vi "Untitled [Tset].vi"() -> ()   [LabVIEW 2012]
uses:
  <vilib>/Analysis/baseanly.llb/Real Dot Product.vi
  <vilib>/Analysis/NI_AALBase.lvlib
panel:
  out "XY Graph":cluster{"Y":dbl[], "Y":dbl[]}[](graph)
  out "Waveform Chart 5":dynamicdata(graph)
  out "Waveform Chart 4":dbl[](graph)
  out "output array":dbl[](array[numeric])
  out "Waveform Chart 3":dbl(graph)
  out "Waveform Chart 2":dynamicdata(graph)
  out "X速率(cm/s)":dbl
  out "Waveform Chart":dbl(graph)
  in  "退出程序":bool caption="停止电机 2"
  out "x/y":dbl
  out "Y偏移量 (cm)":dbl
  out "X偏移量 (cm)":dbl
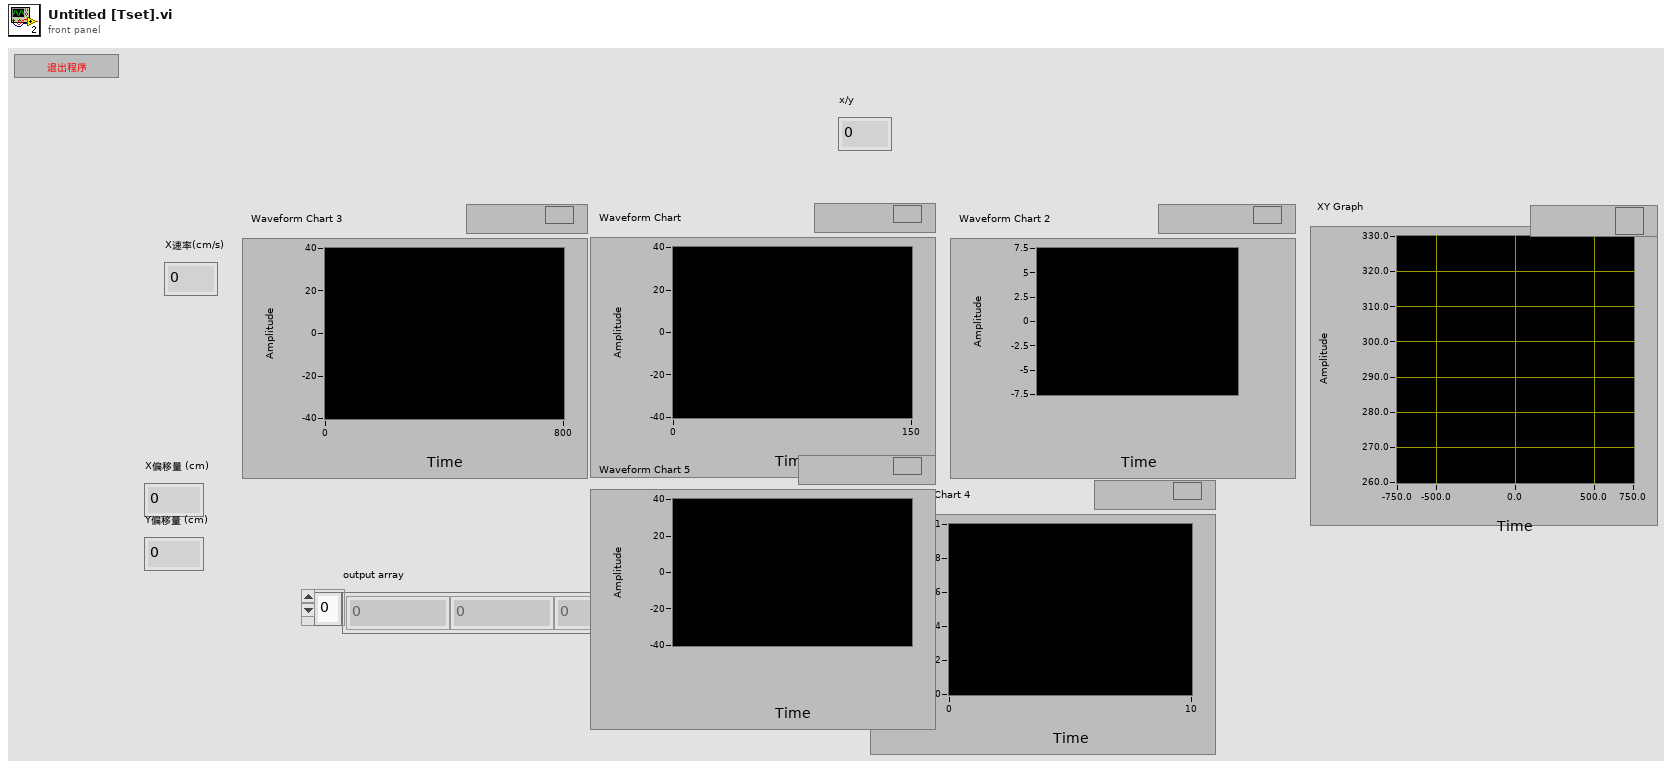
[diagram p1: front panel]
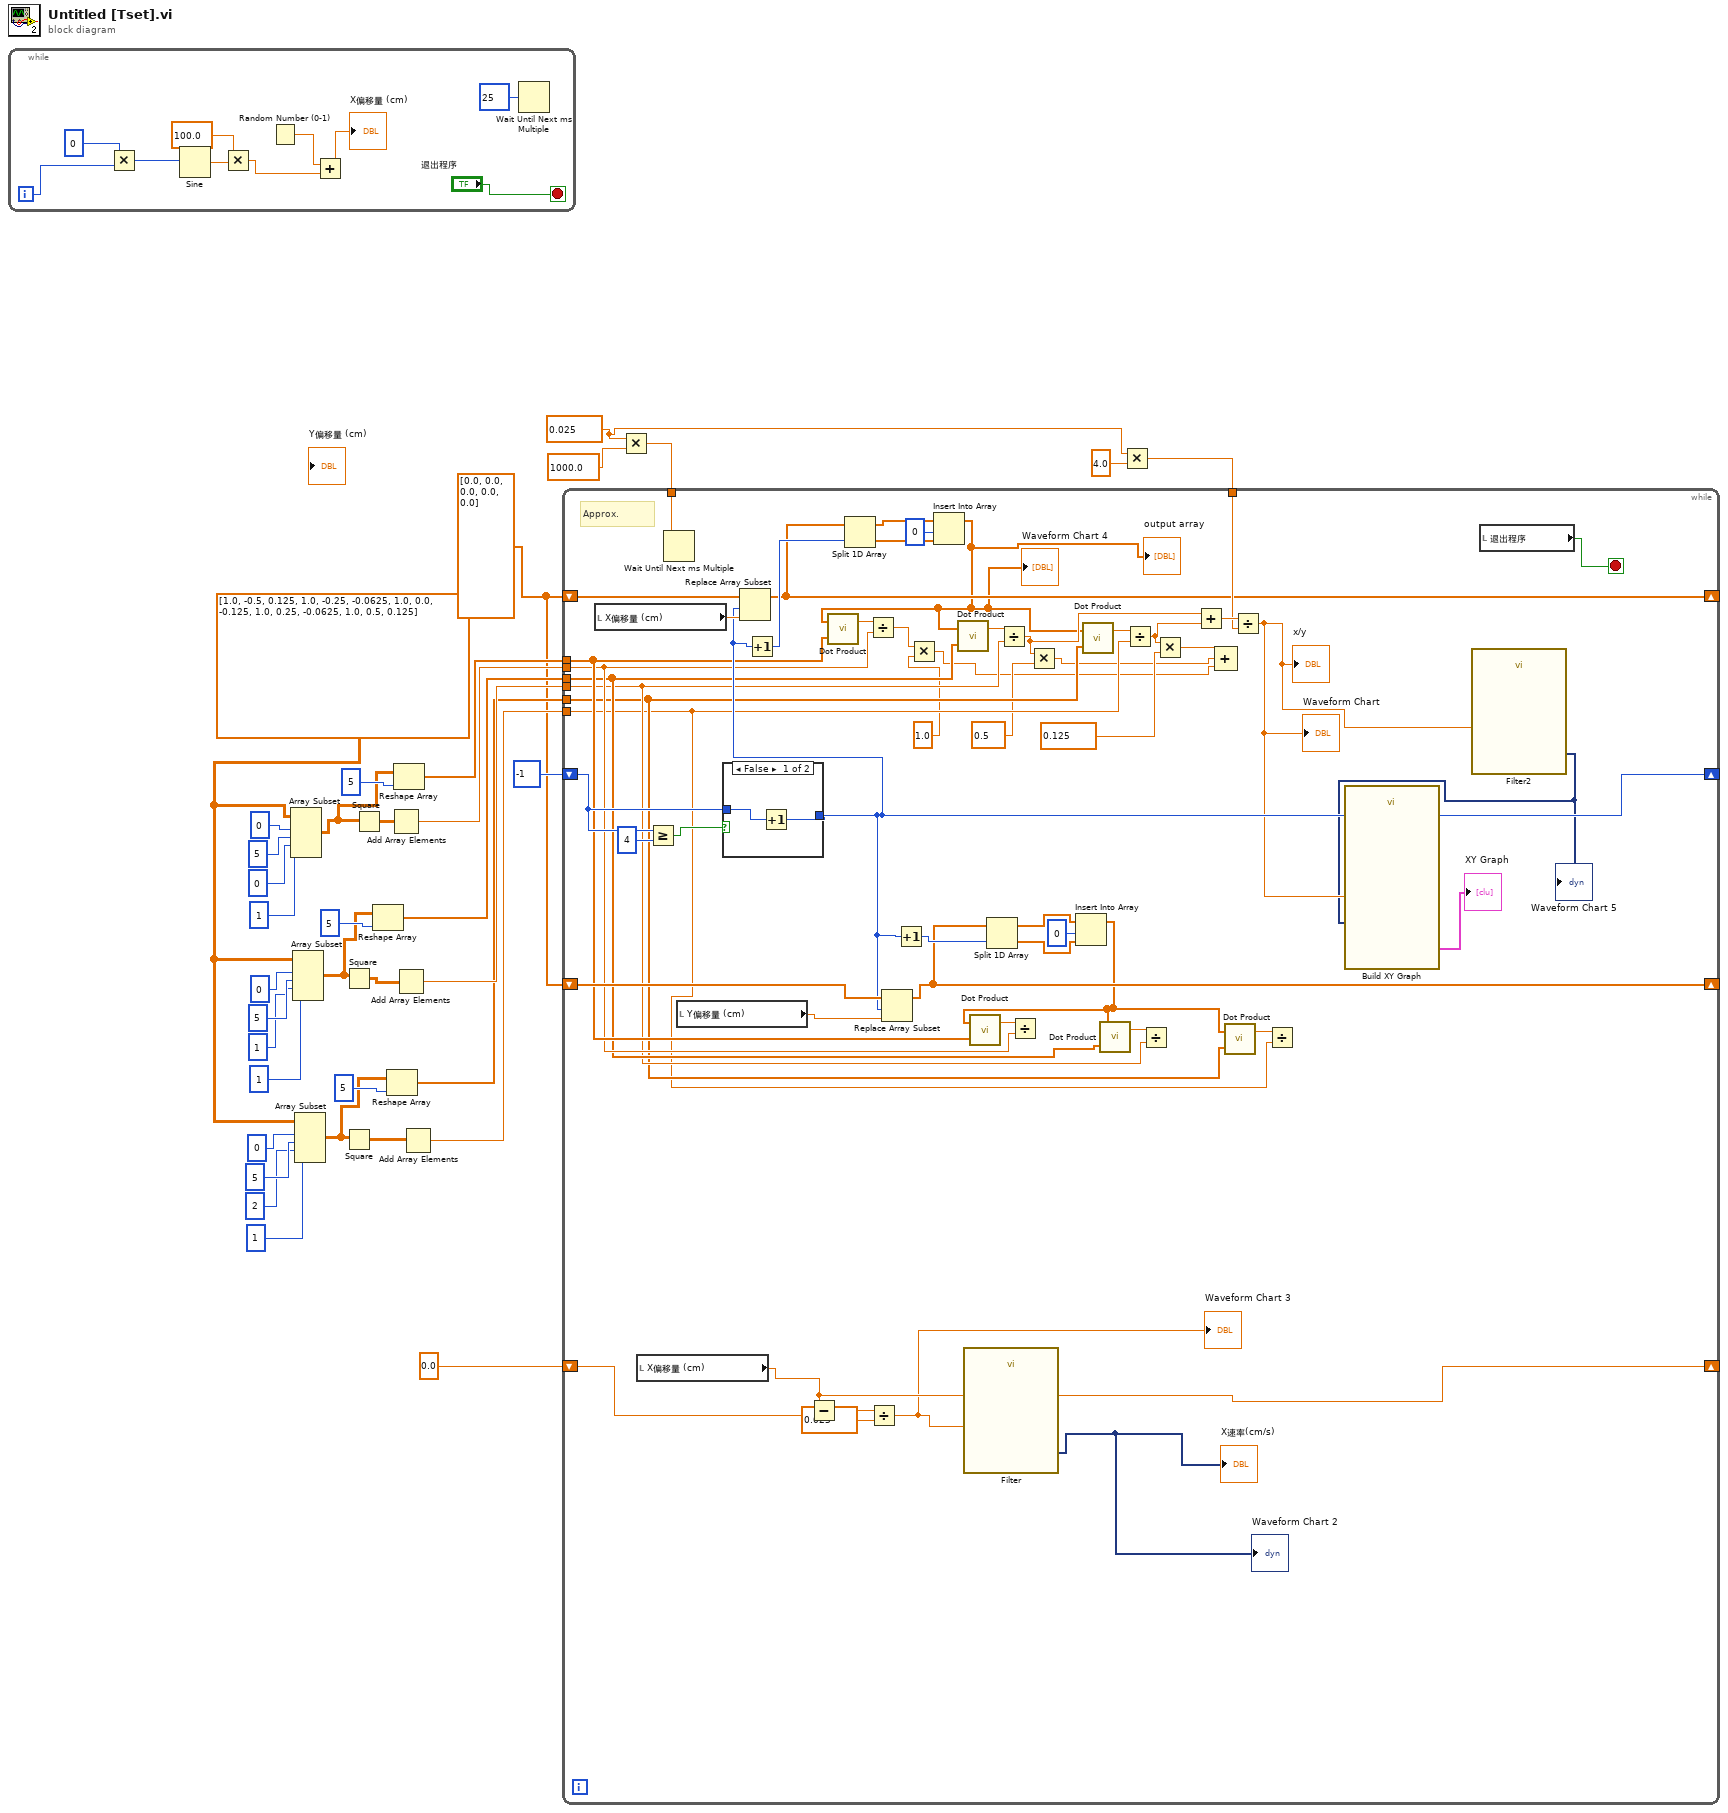
[diagram p0: block diagram]
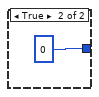
[diagram p2: hidden frame]
diagram:
  w3 = 0.025
  w20 = dbl[][] [[1.0, -0.5, 0.125], [1.0, -0.25, -0.0625], [1.0, 0.0, -0.125], [1.0, 0.25, -0.0625], [1.0, 0.5, 0.125]]
  w7 = dbl[] [0.0, 0.0, 0.0, 0.0, 0.0]
  n1 = while {
    i -> [w43]
    stop <- "退出程序" stop-if-true
    n2 = Multiply(x=0, y=w43) -> (x*y=w40:i32)
    n3 = Sine(x=w40) -> (sin(x)=w39:dbl)
    n4 = Multiply(x=100.0, y=w39) -> (x*y=w37:dbl)
    n5 = Random Number (0-1)() -> (number: 0 to 1=w44:dbl)
    n6 = Add(x=w44, y=w37) -> (x+y=→"X偏移量 (cm)":dbl)
    n7 = Wait Until Next ms Multiple(millisecond multiple=u32 25) -> ()  [unwired: 1 out]
  }
  n8 = Array Subset(array=w20, index (row)=0 ("index"), length (row)=5 ("length"), index (col)=0 ("index"), length (col)=1 ("length")) -> (w18:dbl[][])
  n9 = Array Subset(array=w20, index (row)=0 ("index"), length (row)=5 ("length"), index (col)=1 ("index"), length (col)=1 ("length")) -> (w14:dbl[][])
  n10 = Array Subset(array=w20, index (row)=0 ("index"), length (row)=5 ("length"), index (col)=2 ("index"), length (col)=1 ("length")) -> (w10:dbl[][])
  n11 = Square(x=w14) -> (x^2=w22:dbl[][])
  n12 = Square(x=w10) -> (x^2=w21:dbl[][])
  n13 = Square(x=w18) -> (x^2=w23:dbl[][])
  n14 = Reshape Array(w14, 5 ("dimension size")) -> (w13:dbl[])
  n15 = Reshape Array(w10, 5 ("dimension size")) -> (w9:dbl[])
  n16 = Add Array Elements(numeric array=w23) -> (sum=w16:dbl)
  n17 = Reshape Array(w18, 5 ("dimension size")) -> (w17:dbl[])
  n18 = Add Array Elements(numeric array=w22) -> (sum=w12:dbl)
  n19 = Add Array Elements(numeric array=w21) -> (sum=w8:dbl)
  n20 = Multiply(x=w3, y=1000.0) -> (x*y=w5:dbl)
  n21 = Multiply(x=w3, y=4.0) -> (x*y=w1:dbl)
  n22 = while {
    shift-right: [w51] -> _
    shift-left: w7 -> [w99]
    shift-right: [w85] -> _
    shift-left: -1 -> [w95]
    tunnel: w17 -> [w78]
    tunnel: w16 -> [w77]
    tunnel: w13 -> [w76]
    tunnel: w12 -> [w74]
    tunnel: w9 -> [w72]
    tunnel: w8 -> [w71]
    shift-right: [w83] -> _
    shift-left: w7 -> [w86]
    tunnel: w5 -> [w59]
    tunnel: w1 -> [w58]
    shift-right: [w55] -> _
    shift-left: 0.0 -> [w56]
    stop <- w100 stop-if-true
    # "Approx."
    n23 = local read "X偏移量 (cm)"() -> (w98:dbl)
    n24 = local read "X偏移量 (cm)"() -> (w55:dbl)
    n25 = Greater Or Equal?(x=w95, y=4) -> (x >= y?=w96:bool)
    n26 = Wait Until Next ms Multiple(millisecond multiple=w59) -> ()  [unwired: 1 out]
    n27 = local read "Y偏移量 (cm)"() -> (w87:dbl)
    n28 = case shown="False" w96 {
      tunnel: [w101 0] -> w85
      tunnel: w95 -> [w102 _]
      frame False {
        n29 = Increment(x=w102) -> (x+1=w101:i32)
      }
      frame True {
      }
    }
    n30 = Replace Array Subset(array=w99, new element=w98, index=w85) -> (w51:dbl[])
    n31 = Increment(x=w85) -> (x+1=w91:i32)
    n32 = Subtract(x=w55, y=w56) -> (x-y=w57:dbl)
    n33 = Split 1D Array(array=w51, index=w91) -> (first subarray=w89:dbl[], second subarray=w90:dbl[])
    n34 = Divide(x=w57, y=0.025) -> (x/y=w52:dbl)
    "Waveform Chart 3" <- w52
    n35 = Replace Array Subset(array=w86, new element=w87, index=w85) -> (w83:dbl[])
    n36 = Increment(x=w85) -> (x+1=w84:i32)
    n37 = Insert Into Array(array=w89, index=0, new element=w90) -> (w50:dbl[])
    "output array" <- w50
    "Waveform Chart 4" <- w50
    n38 = call-poly <vilib>:"Dot Product.vi"("Y Vector"=w78, "X Vector"=w50) -> ("X * Y"=w94:dbl)  [unwired: 1 out]
    n39 = Divide(x=w94, y=w77) -> (x/y=w69:dbl)
    n40 = Multiply(x=w69, y=1.0) -> (x*y=w63:dbl)
    n41 = call-poly <vilib>:"Dot Product.vi"("Y Vector"=w76, "X Vector"=w50) -> ("X * Y"=w93:dbl)  [unwired: 1 out]
    n42 = call "Filter"("Signal"=w52) -> ("Filtered Signal"=→"X速率(cm/s)" →"Waveform Chart 2":dynamicdata)  [unwired: 9 in, 1 out]
    n43 = Split 1D Array(array=w83, index=w84) -> (first subarray=w82:dbl[], second subarray=w81:dbl[])
    n44 = Divide(x=w93, y=w74) -> (x/y=w62:dbl)
    n45 = Multiply(x=w62, y=0.5) -> (x*y=w64:dbl)
    n46 = Insert Into Array(array=w82, index=0, new element=w81) -> (w73:dbl[])
    n47 = call-poly <vilib>:"Dot Product.vi"("Y Vector"=w78, "X Vector"=w73) -> ("X * Y"=w79:dbl)  [unwired: 1 out]
    n48 = Divide(x=w79, y=w77) -> ()  [unwired: 1 out]
    n49 = call-poly <vilib>:"Dot Product.vi"("Y Vector"=w72, "X Vector"=w50) -> ("X * Y"=w92:dbl)  [unwired: 1 out]
    n50 = call-poly <vilib>:"Dot Product.vi"("Y Vector"=w76, "X Vector"=w73) -> ("X * Y"=w75:dbl)  [unwired: 1 out]
    n51 = Divide(x=w92, y=w71) -> (x/y=w61:dbl)
    n52 = Divide(x=w75, y=w74) -> ()  [unwired: 1 out]
    n53 = Multiply(x=w61, y=0.125) -> (x*y=w65:dbl)
    n54 = Add(x=w62, y=w61) -> (x+y=w60:dbl)
    n55 = Compound Arithmetic op=ADD(w65, w64, w63) -> ()  [unwired: 1 out]
    n56 = call-poly <vilib>:"Dot Product.vi"("Y Vector"=w72, "X Vector"=w73) -> ("X * Y"=w70:dbl)  [unwired: 1 out]
    n57 = Divide(x=w60, y=w58) -> (x/y=w48:dbl)
    "x/y" <- w48
    "Waveform Chart" <- w48
    n58 = Divide(x=w70, y=w71) -> ()  [unwired: 1 out]
    n59 = call "Filter2"("Signal"=w48) -> ("Filtered Signal"=w47:dynamicdata)  [unwired: 9 in, 1 out]
    "Waveform Chart 5" <- w47
    n60 = call "Build XY Graph"("Y Input"=w47, "X Input"=w48) -> ("XY Graph"=→"XY Graph":cluster{"Y":dbl[], "Y":dbl[]}[])  [unwired: 3 in, 6 out]
    n61 = local read "退出程序"() -> (w100:bool)
  }
